vi "ToUppercase.vi"() -> ()   [LabVIEW 2022 SP3]
panel:
  out "all upper case string":string[](array[string])
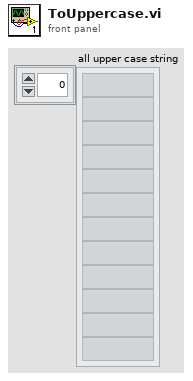
[diagram p1: front panel]
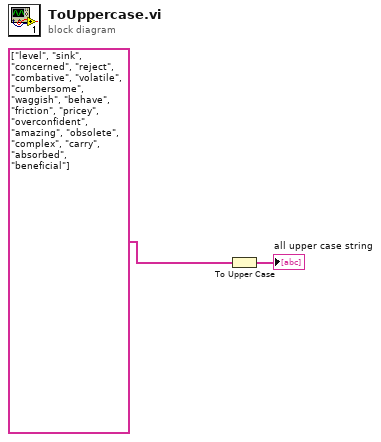
[diagram p0: block diagram]
diagram:
  n1 = To Upper Case(1:string[] ["level", "sink", "concerned", "reject", "combative", "volatile", "cumbersome", "waggish", "behave", "friction", "pricey", "overconfident", "amazing", "obsolete", "complex", "carry", "absorbed", "beneficial"] ("Word List")) -> (0:→"all upper case string":string[])
